vi "filter_mean_last_n_values.vi"(0 "x in":dbl[](array[numeric]), 7 "y in":dbl[](array[numeric]), 11 "z in":dbl[](array[numeric]), 13 "last n values":i32) -> (4 "x out":dbl, 8 "y out":dbl, 15 "z out":dbl)   [LabVIEW 2023]
uses:
  <vilib>/Analysis/NI_AALBase.lvlib
  <vilib>/Analysis/baseanly.llb/Mean (DBL).vi
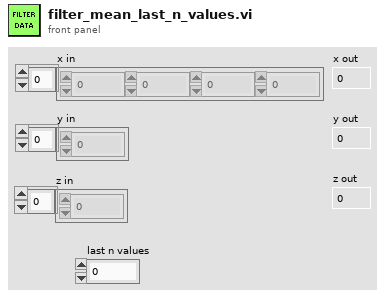
[diagram p1: front panel]
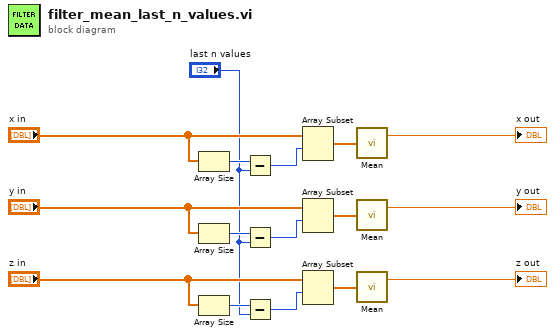
[diagram p0: block diagram]
diagram:
  n1 = Array Size(array="x in") -> (size(s)=w15:i32)
  n2 = Array Size(array="y in") -> (size(s)=w9:i32)
  n3 = Array Size(array="z in") -> (size(s)=w7:i32)
  n4 = Subtract(x=w15, y="last n values") -> (x-y=w14:i32)
  n5 = Subtract(x=w9, y="last n values") -> (x-y=w10:i32)
  n6 = Subtract(x=w7, y="last n values") -> (x-y=w6:i32)
  n7 = Array Subset(array="x in", index=w14) -> (w13:dbl[])  [unwired: 1 in]
  n8 = Array Subset(array="y in", index=w10) -> (w11:dbl[])  [unwired: 1 in]
  n9 = Array Subset(array="z in", index=w6) -> (w5:dbl[])  [unwired: 1 in]
  n10 = call-poly <vilib>:"Mean.vi"("X"=w13) -> ("mean"=→"x out":dbl)  [unwired: 1 out]
  n11 = call-poly <vilib>:"Mean.vi"("X"=w11) -> ("mean"=→"y out":dbl)  [unwired: 1 out]
  n12 = call-poly <vilib>:"Mean.vi"("X"=w5) -> ("mean"=→"z out":dbl)  [unwired: 1 out]
